vi "emi_Standalone or Called.vi"(11 "error in (no error)":errorcluster) -> (8 "Called":bool, 15 "error out":errorcluster)   [LabVIEW 2010]
doc: "If the VI where this is placed was started directly by user, it returns TRUE. If it is called by another VI it returns FALSE.\n\nIntended use: Being able to create code specificaly for testing/runnig a vi as standalone as oposed to its normal configuration.\n\nOn Error: No change"
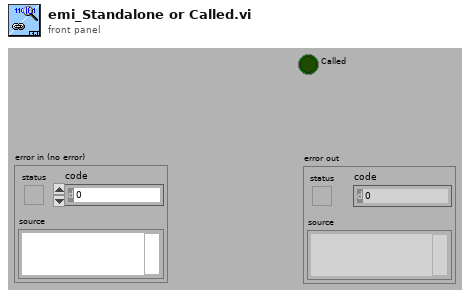
[diagram p1: front panel]
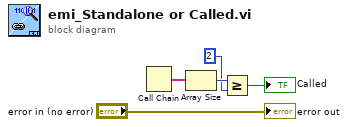
[diagram p0: block diagram]
diagram:
  n1 = Call Chain() -> (call chain=w4:string[])
  n2 = Array Size(array=w4) -> (size(s)=w3:i32)
  n3 = Greater Or Equal?(x=w3, y=2) -> (x >= y?=→"Called":bool)
  "error out" <- "error in (no error)"
